vi "ClusterToControls.vi"(11 "Path File Data":T1 {"RobotNeeded"."SlowSpeed" format="%#_13g"; "RobotNeeded"."SlowDistanceAtEnd" format="%#_13g"; "RobotNeeded"."Speed/Curve" format="%#_13g"}) -> (3 "Path (px)":cluster{i32, i32}[](array[cluster]))   [LabVIEW 2019]
uses:
  Dawgma Programming Library/Controls/PurePursuit/PathFileData.ctl
  Dawgma Programming Library/Controls/PurePursuit/RobotNeededPathData.ctl
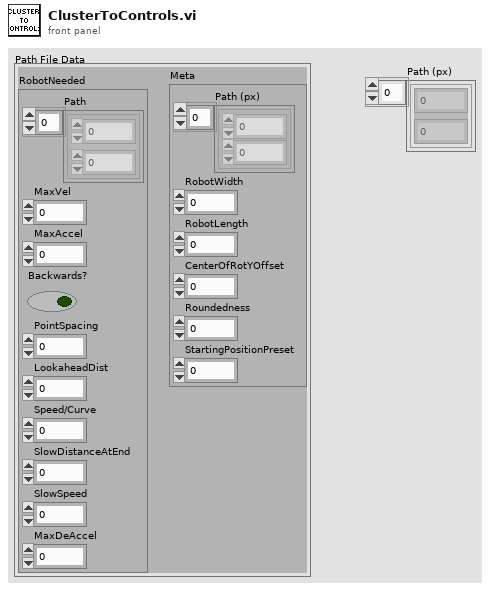
[diagram p1: front panel]
types:
  T1 = typedef "PathFileData.ctl" = cluster{"RobotNeeded":T2, "Meta":cluster{"Path (px)":cluster{i32, i32}[], "RobotWidth":dbl, "RobotLength":dbl, "CenterOfRotYOffset":dbl, "Roundedness":dbl, "StartingPositionPreset":u32}}
  T2 = typedef "RobotNeededPathData.ctl" = cluster{"Path":cluster{dbl, dbl}[], "MaxVel":dbl, "MaxAccel":dbl, "Backwards?":bool, "PointSpacing":dbl, "LookaheadDist":dbl, "Speed/Curve":dbl, "SlowDistanceAtEnd":dbl, "SlowSpeed":dbl, "MaxDeAccel":dbl}
  T3 = cluster{"Path (px)":cluster{i32, i32}[], "RobotWidth":dbl, "RobotLength":dbl, "CenterOfRotYOffset":dbl, "Roundedness":dbl, "StartingPositionPreset":u32}
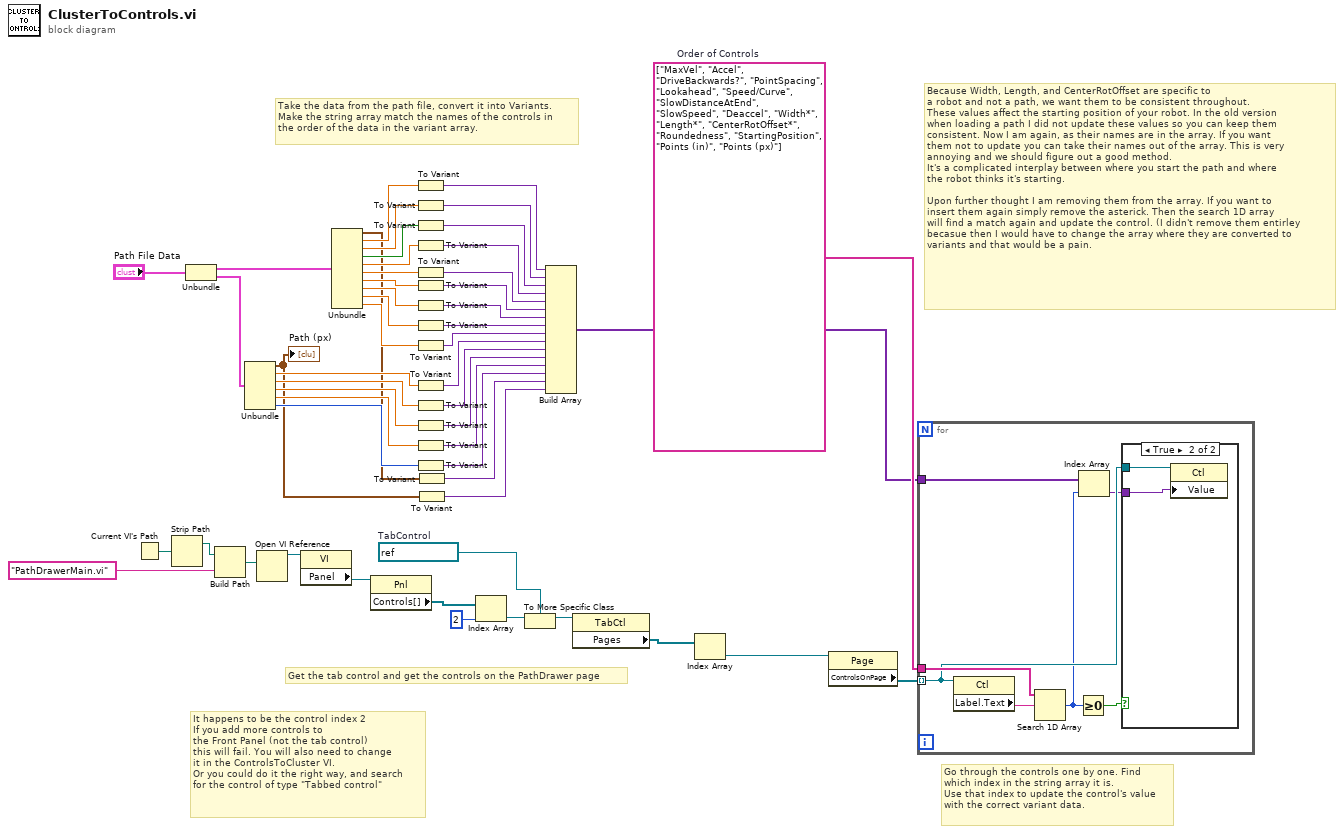
[diagram p0: block diagram]
diagram:
  w45 = string[] ["MaxVel", "Accel", "DriveBackwards?", "PointSpacing", "Lookahead", "Speed/Curve", "SlowDistanceAtEnd", "SlowSpeed", "Deaccel", "Width*", "Length*", "CenterRotOffset*", "Roundedness", "StartingPosition", "Points (in)", "Points (px)"]  # Order of Controls
  w50 = refnum<vi> refnum  # TabControl
  # "Take the data from the path file, convert it into Variants.\nMake the string array match the names of the controls in\nthe order of the data in the variant array."
  # "It happens to be the control index 2\nIf you add more controls to\nthe Front Panel (not the tab control)\nthis will fail. You will also need to change\nit in the ControlsToCluster VI.\nOr you could do it the right way, and search\nfor the control of type \"Tabbed control\""
  # "Because Width, Length, and CenterRotOffset are specific to\na robot and not a path, we want them to be consistent throughout.\nThese values affect the starting position of your robot. In the old version\nwhen loading a path I did not update these values so you can keep them\nconsistent. Now I am again, as their names are in the array. If you want\nthem not to update you can take their names out of the array. This is very\nannoying and we should figure out a good method.\nIt's a complicated interplay between where you start the path and where\nthe robot thinks it's starting. \n\nUpon further thought I am removing them from the array. If you want to\ninsert them again simply remove the asterick. Then the search 1D array\nwill find a match again and update the control. (I didn't remove them entirley\nbecasue then I would have to change the array where they are converted to \nvariants and that would be a pain."
  # "Go through the controls one by one. Find\nwhich index in the string array it is.\nUse that index to update the control's value\nwith the correct variant data."
  # "Get the tab control and get the controls on the PathDrawer page"
  n1 = Current VI's Path() -> (path=w43:path)
  n2 = Strip Path(path=w43) -> (stripped path=w42:path)  [unwired: 1 out]
  n3 = Unbundle("Path File Data") -> ("RobotNeeded"=w24:T2, "Meta"=w25:T3)
  n4 = Build Path(base path=w42, name or relative path="PathDrawerMain.vi") -> (appended path=w40:path)
  n5 = Unbundle(w25) -> ("Path (px)"=w8:cluster{i32, i32}[], "RobotWidth"=w14:dbl, "RobotLength"=w13:dbl, "CenterOfRotYOffset"=w12:dbl, "Roundedness"=w11:dbl, "StartingPositionPreset"=w10:u32)
  "Path (px)" <- w8
  n6 = Open VI Reference(vi path=w40) -> (vi reference=w39:refnum<vi>)  [unwired: 5 in, 1 out]
  n7 = property class="VI"(reference=w39) -> ("Panel"=w44:refnum<vi>)  [unwired: 1 in, 2 out]
  n8 = Unbundle(w24) -> ("Path"=w9:cluster{dbl, dbl}[], "MaxVel"=w23:dbl, "MaxAccel"=w22:dbl, "Backwards?"=w21:bool, "PointSpacing"=w20:dbl, "LookaheadDist"=w19:dbl, "Speed/Curve"=w18:dbl, "SlowDistanceAtEnd"=w17:dbl, "SlowSpeed"=w16:dbl, "MaxDeAccel"=w15:dbl)
  n9 = property class="Pnl"(reference=w44) -> ("Controls[]"=w38:refnum<vi>[])  [unwired: 1 in, 2 out]
  n10 = To Variant(anything=w23) -> (Variant=w37:variant)
  n11 = To Variant(anything=w22) -> (Variant=w36:variant)
  n12 = To Variant(anything=w21) -> (Variant=w35:variant)
  n13 = To Variant(anything=w20) -> (Variant=w34:variant)
  n14 = To Variant(anything=w19) -> (Variant=w33:variant)
  n15 = To Variant(anything=w18) -> (Variant=w32:variant)
  n16 = To Variant(anything=w17) -> (Variant=w31:variant)
  n17 = To Variant(anything=w16) -> (Variant=w30:variant)
  n18 = To Variant(anything=w15) -> (Variant=w29:variant)
  n19 = To Variant(anything=w14) -> (Variant=w28:variant)
  n20 = To Variant(anything=w13) -> (Variant=w27:variant)
  n21 = To Variant(anything=w12) -> (Variant=w7:variant)
  n22 = To Variant(anything=w11) -> (Variant=w6:variant)
  n23 = To Variant(anything=w10) -> (Variant=w5:variant)
  n24 = To Variant(anything=w9) -> (Variant=w4:variant)
  n25 = To Variant(anything=w8) -> (Variant=w3:variant)
  n26 = Index Array(array=w38, index=2) -> (element=w49:refnum<vi>)
  n27 = To More Specific Class(target class=w50, reference=w49) -> (specific class reference=w48:refnum<vi>)  [unwired: 1 in, 1 out]
  n28 = Build Array(w37, w36, w35, w34, w33, w32, w31, w30, w29, w28, w27, w7, w6, w5, w4, w3) -> (w1:variant[])
  n29 = property class="TabCtl"(reference=w48) -> ("Pages"=w47:refnum<vi>[])  [unwired: 1 in, 2 out]
  n30 = Index Array(array=w47) -> (element=w46:refnum<vi>)  [unwired: 1 in]
  n31 = property class="Page"(reference=w46) -> ("ControlsOnPage"=w2:refnum<vi>[])  [unwired: 1 in, 2 out]
  n32 = for {
    tunnel: w45 -> [w57]
    tunnel: w2 -> [w55] mode=indexing
    tunnel: w1 -> [w54]
    n33 = property class="Ctl"(reference=w55) -> ("Label.Text"=w58:string)  [unwired: 1 in, 2 out]
    n34 = Search 1D Array(1D array=w57, element=w58) -> (index of element=w52:i32)  [unwired: 1 in]
    n35 = Greater Or Equal To 0?(x=w52) -> (x >= 0?=w56:bool)
    n36 = Index Array(array=w54, index=w52) -> (element=w53:variant)
    n37 = case shown="True" w56 {
      tunnel: w55 -> [_ w60]
      tunnel: w53 -> [_ w59]
      frame False {
      }
      frame True {
        n38 = property class="Ctl"(reference=w60, "Value"=w59) -> ()  [unwired: 1 in, 2 out]
      }
    }
  }
